vi "Wait for Message.vi"(8 "error in":errorcluster, 10 "Timeout":i32 format="%d ms", 11 "Message Waiter in":refnum<class "Message Waiter.lvclass">) -> (0 "error out":errorcluster, 2 "Timed Out":bool, 3 "Message Waiter out":refnum<class "Message Waiter.lvclass">)   [LabVIEW 2020, in "PCANBasic.lvlib" / "Message Waiter.lvclass"]
uses:
  Message Waiter.lvclass
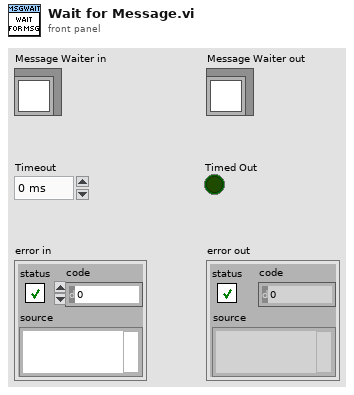
[diagram p1: front panel]
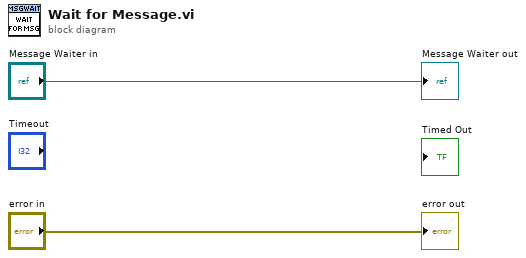
[diagram p0: block diagram]
diagram:
  "error out" <- "error in"
  "Message Waiter out" <- "Message Waiter in"
